vi "Acquisition Message Loop.vi"(8 "error in (no error)":errorcluster, 9 "Data Queue":refnum<queue>, 10 "Data Queue 2":refnum<queue>, 11 "Message Queues":T1) -> (0 "error out":errorcluster)   [LabVIEW 2016, in "Acquisition.lvlib"]
doc: "Message loop for handling messages pertaining to the acquisition of data from the hardware."
uses:
  Acquisition.lvlib
  support/Message Queue/All Message Queues.ctl
  support/Message Queue/Message Cluster.ctl
  Hardware Configuration.ctl
  Acquisition State.ctl
  support/Message Queue/Enqueue Message (Single).vi
  <vilib>/Utility/error.llb/Error Cluster From Error Code.vi
  <vilib>/ErrorRing/Error Ring.xnode
  support/Message Queue/Message Queue.lvlib
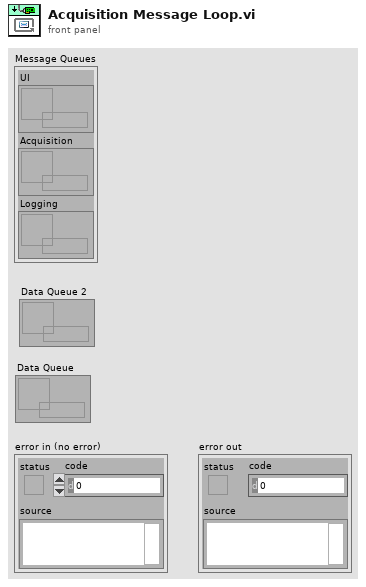
[diagram p1: front panel]
types:
  T1 = typedef "Message Queue.lvlib/All Message Queues.ctl" = cluster{"UI":refnum<queue>, "Acquisition":refnum<queue>, "Logging":refnum<queue>}
  T2 = typedef "Acquisition.lvlib/Hardware Configuration.ctl" = cluster{"DAQmx Input":tag, "Max Input":dbl, "Min Input":dbl, "Sample Rate":dbl, "DAQmx Task":refnum<k21>}
  T3 = typedef "Acquisition.lvlib/Acquisition State.ctl" = enum16{"Idle", "Acquiring"}
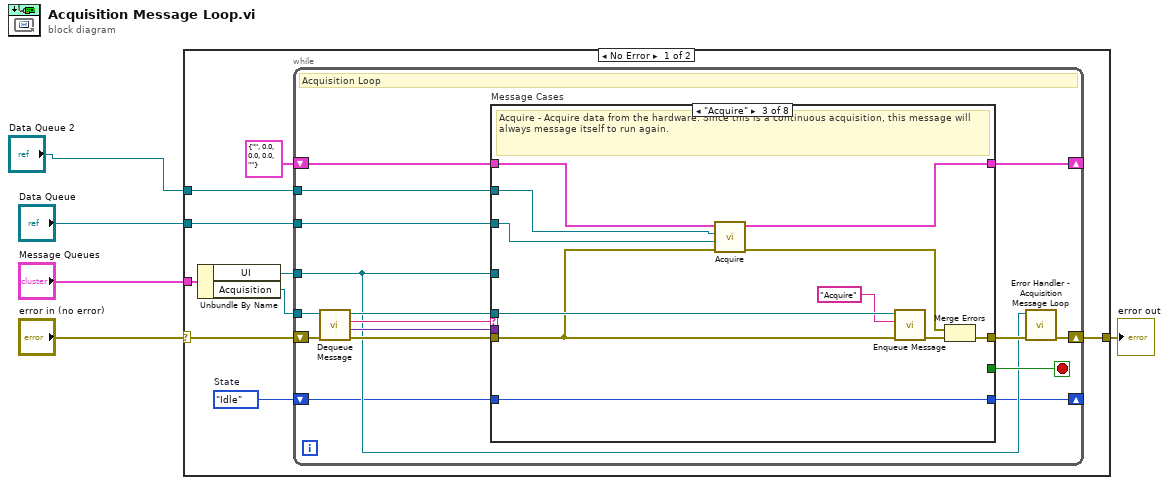
[diagram p0: block diagram]
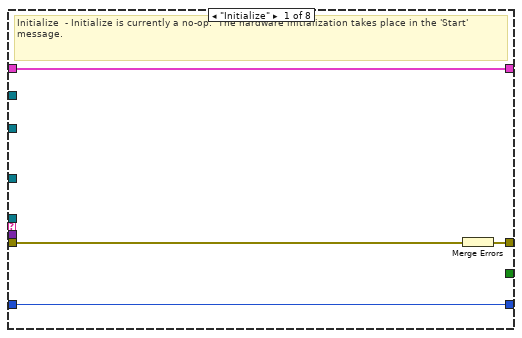
[diagram p2: hidden frame]
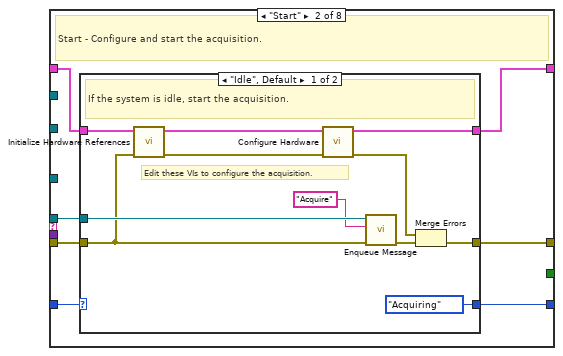
[diagram p3: hidden frame]
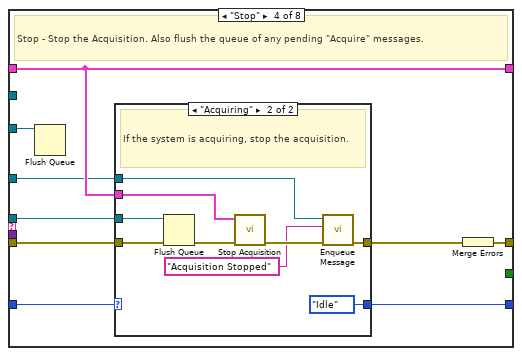
[diagram p5: hidden frame]
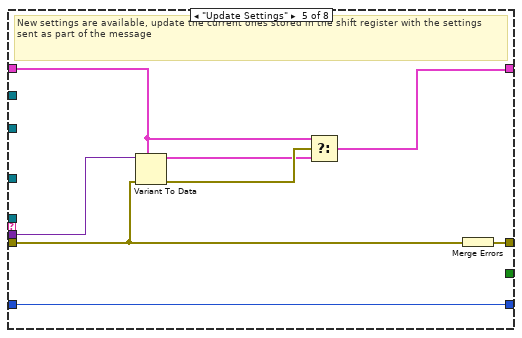
[diagram p7: hidden frame]
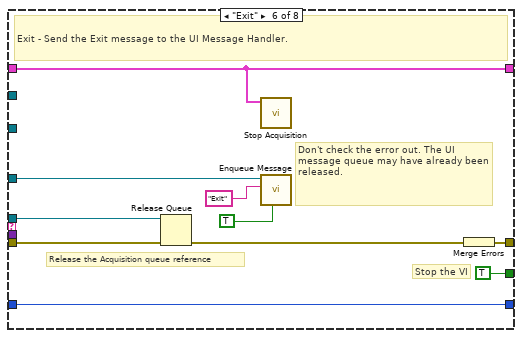
[diagram p8: hidden frame]
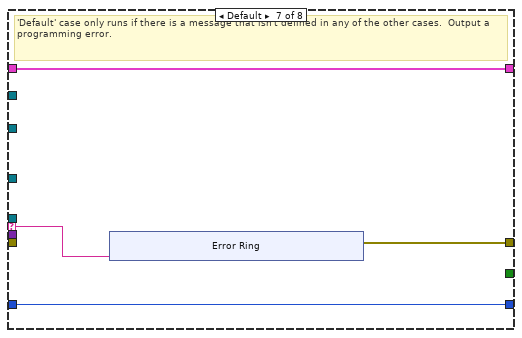
[diagram p9: hidden frame]
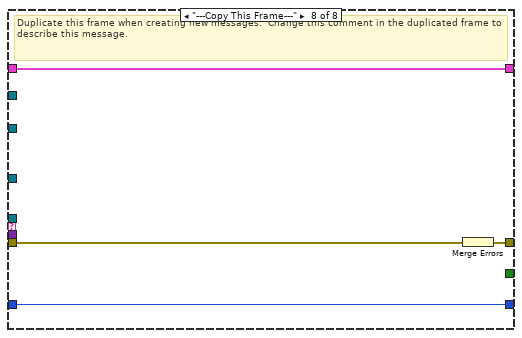
[diagram p10: hidden frame]
diagram:
  n1 = case shown="No Error" "error in (no error)" {
    selector: "error in (no error)" -> [w10 w120]
    tunnel: "Message Queues" -> [w14 _]
    tunnel: [w12 w120] -> w4
    tunnel: "Data Queue 2" -> [w8 _]
    tunnel: "Data Queue" -> [w7 _]
    frame No Error {
      w6 = Acquisition_State."Idle"  # State
      n2 = Unbundle By Name(w14) -> ("UI"=w9:refnum<queue>, "Acquisition"=w13:refnum<queue>)
      n3 = while {
        tunnel: w13 -> [w22]
        shift-right: [w29] -> _
        shift-left: T2 {"DAQmx Input"="", "Max Input"=0.0, "Min Input"=0.0, "Sample Rate"=0.0, "DAQmx Task"=""} ("Data Cluster") -> [w30]
        shift-right: [w18] -> w12
        shift-left: w10 -> [w27]
        tunnel: w9 -> [w17]
        tunnel: w8 -> [w21]
        tunnel: w7 -> [w20]
        shift-right: [w15] -> _
        shift-left: w6 -> [w16]
        stop <- w28 stop-if-true
        # "Acquisition Loop"
        n4 = call "Dequeue Message.vi"("error in (no error)"=w27, "Message Queue"=w22) -> ("error out"=w26:errorcluster, "Message Data"=w24:variant, "Message"=w25:string, "dup Message Queue"=w23:refnum<queue>)  [unwired: 6 in]
        n5 = case "Message Cases" shown="\"Acquire\"" w25 {
          selector: w25 -> [_ _ _ _ _ _ w107 _]
          tunnel: w23 -> [_ w38 w64 w72 _ w97 _ _]
          tunnel: w26 -> [w33 w39 w63 w74 w88 w101 _ w119]
          tunnel: [w34 w41 w66 w75 w94 w103 w106 w117] -> w19
          tunnel: w30 -> [w32 w40 w60 w73 w90 w96 w108 w118]
          tunnel: [w32 w37 w61 w73 w89 w96 w108 w118] -> w29
          tunnel: [_ _ _ _ _ TRUE _ _] -> w28
          tunnel: w24 -> [_ _ _ _ w93 _ _ _]
          tunnel: w17 -> [_ _ _ w71 _ w102 _ _]
          tunnel: w21 -> [_ _ w56 _ _ _ _ _]
          tunnel: w20 -> [_ _ w58 w67 _ _ _ _]
          tunnel: w16 -> [w31 w36 w57 w70 w87 w95 w105 w116]
          tunnel: [w31 w35 w57 w69 w87 w95 w105 w116] -> w15
          frame "Initialize" {
            # "Initialize  - Initialize is currently a no-op.  The hardware initialization takes place in the 'Start' message."
            n6 = Merge Errors(w33) -> (w34:errorcluster)
          }
          frame "Start" {
            # "Start - Configure and start the acquisition."
            n7 = case shown="\"Idle\", Default" w36 {
              selector: w36 -> [_ w53]
              tunnel: [w52 w55] -> w41
              tunnel: w40 -> [w45 w54]
              tunnel: w39 -> [w44 w55]
              tunnel: w38 -> [w50 _]
              tunnel: [w48 w54] -> w37
              tunnel: [Acquisition_State."Acquiring" ("State") w53] -> w35
              frame "Idle", Default {
                # "Edit these VIs to configure the acquisition."
                # "If the system is idle, start the acquisition."
                n8 = call "Initialize Hardware References.vi"("error in (no error)"=w44, "Hardware Resources in"=w45) -> ("error out"=w42:errorcluster, "Hardware Resources out"=w43:T2)  [unwired: 8 in]
                n9 = call "Configure Hardware.vi"("error in (no error)"=w42, "Hardware Resources in"=w43) -> ("error out"=w49:errorcluster, "Hardware Resources out"=w48:T2)  [unwired: 8 in]
                n10 = call-poly "Enqueue Message.vi"("error in (no error)"=w44, "Message"="Acquire", "Message Queue"=w50) -> ("error out"=w51:errorcluster)  [unwired: 7 in, 1 out]
                n11 = Merge Errors(w49, w51) -> (w52:errorcluster)
              }
              frame "Acquiring" {
                # "The system is already acquiring. Ignore the \"Start\" message."
              }
            }
          }
          frame "Acquire" {
            # "Acquire - Acquire data from the hardware. Since this is a continuous acquisition, this message will always message itself to run again."
            n12 = call "Acquire.vi"("error in (no error)"=w63, "Data Queue"=w58, "Data Queue 2"=w56, "Hardware Resources in"=w60) -> ("error out"=w62:errorcluster, "Hardware Resources out"=w61:T2)  [unwired: 6 in]
            n13 = call-poly "Enqueue Message.vi"("error in (no error)"=w63, "Message"="Acquire", "Message Queue"=w64) -> ("error out"=w65:errorcluster)  [unwired: 7 in, 1 out]
            n14 = Merge Errors(w62, w65) -> (w66:errorcluster)
          }
          frame "Stop" {
            # "Stop - Stop the Acquisition. Also flush the queue of any pending \"Acquire\" messages."
            n15 = Flush Queue(queue=w67) -> ()  [unwired: 1 in, 3 out]
            n16 = case shown="\"Acquiring\"" w70 {
              selector: w70 -> [w77 _]
              tunnel: w74 -> [w76 w86]
              tunnel: w73 -> [_ w85]
              tunnel: w72 -> [_ w83]
              tunnel: w71 -> [_ w82]
              tunnel: [w77 Acquisition_State."Idle" ("State")] -> w69
              tunnel: [w76 w80] -> w68
              frame "Idle", Default {
                # "The system is already idle. Ignore the \"Stop\" message."
              }
              frame "Acquiring" {
                # "If the system is acquiring, stop the acquisition."
                n17 = Flush Queue(queue=w83, error in (no error)=w86) -> (error out=w84:errorcluster)  [unwired: 2 out]
                n18 = call "Stop Acquisition.vi"("error in (no error)"=w84, "Hardware Resources in"=w85) -> ("error out"=w81:errorcluster)  [unwired: 9 in]
                n19 = call-poly "Enqueue Message.vi"("error in (no error)"=w81, "Message"="Acquisition Stopped", "Message Queue"=w82) -> ("error out"=w80:errorcluster)  [unwired: 7 in, 1 out]
              }
            }
            n20 = Merge Errors(w68) -> (w75:errorcluster)
          }
          frame "Update Settings" {
            # "New settings are available, update the current ones stored in the shift register with the settings sent as part of the message"
            n21 = Variant To Data(error in=w88, type=w90, Variant=w93) -> (data=w91:T2, error out=w92:errorcluster)
            n22 = Select(t=w90, s=w92, f=w91) -> (s? t:f=w89:T2)
            n23 = Merge Errors(w88) -> (w94:errorcluster)
          }
          frame "Exit" {
            # "Don't check the error out. The UI message queue may have already been released."
            # "Release the Acquisition queue reference"
            # "Stop the VI"
            # "Exit - Send the Exit message to the UI Message Handler."
            n24 = Release Queue(queue=w97, error in (no error)=w101) -> (error out=w98:errorcluster)  [unwired: 1 in, 2 out]
            n25 = call "Stop Acquisition.vi"("Hardware Resources in"=w96) -> ()  [unwired: 10 in, 1 out]
            n26 = call-poly "Enqueue Message.vi"("Priority Message? (F)"=TRUE, "Message"="Exit", "Message Queue"=w102) -> ()  [unwired: 7 in, 2 out]
            n27 = Merge Errors(w98) -> (w103:errorcluster)
          }
          frame Default {
            # "'Default' case only runs if there is a message that isn't defined in any of the other cases.  Output a programming error."
            n28 = xnode "Error Ring"("parameter 0"=w107) -> ("error out"=w106:errorcluster)
          }
          frame "---Copy This Frame---" {
            # "Duplicate this frame when creating new messages.  Change this comment in the duplicated frame to describe this message."
            n29 = Merge Errors(w119) -> (w117:errorcluster)
          }
        }
        n30 = call "Error Handler - Acquisition Message Loop.vi"("error in (no error)"=w19, "Message Queue"=w17) -> ("dup error in"=w18:errorcluster)  [unwired: 8 in, 1 out]
      }
    }
    frame Error {
    }
  }
  "error out" <- w4
